vi "set ZMQ timeouts - low level.vi"(8 "error in (no error)":errorcluster, 10 "ZMQ new Timeouts in":T1={"SNDTIMEO"=-1, "RCVTIMEO"=-1}, 11 "zmq_socket in":refnum<class "zmq_socket.lvclass">) -> (0 "error out":errorcluster, 2 "ZMQ new Timeouts out":T1, 3 "zmq_socket out":refnum<class "zmq_socket.lvclass">)   [LabVIEW 2018, in "LV2Julia_core.lvlib"]
uses:
  LV2Julia_core.lvlib
  <vilib>/addons/zeromq/zmq_socket.lvclass
  ZMQ timeouts.ctl
  <vilib>/addons/zeromq/socket_options.ctl
  <vilib>/addons/zeromq/zmq_getsocketopt_int.vi
  <vilib>/addons/zeromq/zeromq.lvlib
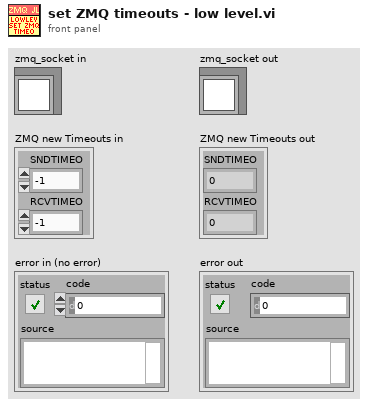
[diagram p1: front panel]
types:
  T1 = typedef "LV2Julia_core.lvlib/ZMQ timeouts.ctl" = cluster{"SNDTIMEO":i32, "RCVTIMEO":i32}
  T2 = typedef "zeromq.lvlib/socket_options.ctl" = enum8{"NONE", "ZMQ_HWM", "<2>", "ZMQ_SWAP", "ZMQ_AFFINITY", "ZMQ_IDENTITY", "ZMQ_SUBSCRIBE", "ZMQ_UNSUBSCRIBE", "ZMQ_RATE", "ZMQ_RECOVERY_IVL", "ZMQ_MCAST_LOOP", "ZMQ_SNDBUF", "ZMQ_RCVBUF", "ZMQ_RCVMORE", "ZMQ_FD", "ZMQ_EVENTS", "ZMQ_TYPE", "ZMQ_LINGER", "ZMQ_RECONNECT_IVL", "ZMQ_BACKLOG", "ZMQ_RECOVERY_IVL_MSEC", "ZMQ_RECONNECT_IVL_MAX", "ZMQ_MAXMSGSIZE", "ZMQ_SNDHWM", "ZMQ_RCVHWM", "ZMQ_MULTICAST_HOPS", "<26>", "ZMQ_RCVTIMEO", "ZMQ_SNDTIMEO", "<29>", "<30>", "ZMQ_IPV4ONLY", "ZMQ_LAST_ENDPOINT", "ZMQ_ROUTER_MANDATORY", "ZMQ_TCP_KEEPALIVE", "ZMQ_TCP_KEEPALIVE_CNT", "ZMQ_TCP_KEEPALIVE_IDLE", "ZMQ_TCP_KEEPALIVE_INTVL", "ZMQ_TCP_ACCEPT_FILTER", "ZMQ_DELAY_ATTACH_ON_CONNECT", "ZMQ_XPUB_VERBOSE"}
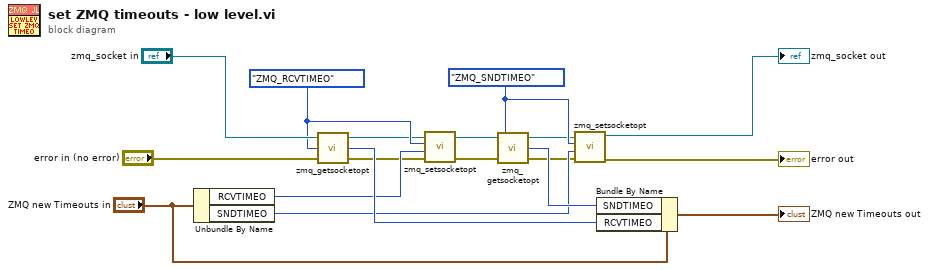
[diagram p0: block diagram]
diagram:
  w7 = socket_options."ZMQ_SNDTIMEO" ("option")
  w12 = socket_options."ZMQ_RCVTIMEO" ("option")
  n1 = Unbundle By Name("ZMQ new Timeouts in") -> ("RCVTIMEO"=w10:i32, "SNDTIMEO"=w11:i32)
  n2 = call-poly <vilib>:"zmq_getsocketopt.vi"("error in"="error in (no error)", "option"=w12, "socket in"="zmq_socket in") -> ("error out"=w1:errorcluster, "value"=w15:i32, "socket out"=w2:refnum<class "zmq_socket.lvclass">)
  n3 = call <vilib>:"zmq_setsocketopt.vi"("error in"=w1, "value"=w10, "option"=w12, "socket in"=w2) -> ("error out"=w6:errorcluster, "socket out"=w5:refnum<class "zmq_socket.lvclass">)  [unwired: 2 in]
  n4 = call-poly <vilib>:"zmq_getsocketopt.vi"("error in"=w6, "option"=w7, "socket in"=w5) -> ("error out"=w4:errorcluster, "value"=w16:i32, "socket out"=w3:refnum<class "zmq_socket.lvclass">)
  n5 = call <vilib>:"zmq_setsocketopt.vi"("error in"=w4, "value"=w11, "option"=w7, "socket in"=w3) -> ("error out"=→"error out":errorcluster, "socket out"=→"zmq_socket out":refnum<class "zmq_socket.lvclass">)  [unwired: 2 in]
  n6 = Bundle By Name(cluster="ZMQ new Timeouts in", "SNDTIMEO"=w16, "RCVTIMEO"=w15) -> (→"ZMQ new Timeouts out":T1)
